vi "EvaluateBooleanLogic.vi"() -> ()   [LabVIEW 2010]
panel:
  out "lol":bool
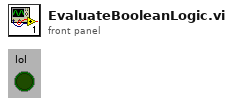
[diagram p1: front panel]
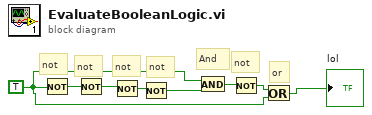
[diagram p0: block diagram]
diagram:
  w2 = TRUE
  # "or"
  # "not"
  # "And"
  # "not"
  # "not"
  # "not"
  # "not"
  n1 = Not(x=w2) -> (.not. x?=w8:bool)
  n2 = Not(x=w8) -> (.not. x?=w7:bool)
  n3 = Not(x=w7) -> (.not. x?=w6:bool)
  n4 = Not(x=w6) -> (.not. x?=w5:bool)
  n5 = And(x=w2, y=w5) -> (x .and. y?=w4:bool)
  n6 = Not(x=w4) -> (.not. x?=w3:bool)
  n7 = Or(x=w3, y=w2) -> (x .or. y?=→"lol":bool)
